vi "Send Control Drag Ended.vi"(0 "Message Enqueuer in":refnum<class "Message Enqueuer.lvclass">, 5 "CtlRef":refnum<vi>, 7 "Time":u32, 9 "Result":enum16{"Drop Cancel", "Drop Move", "Drop Copy"}(ring)) -> (4 "Filtered EventDataMessage":refnum<class "ControlDragEndedMsg.lvclass">, 15 "error out":errorcluster)   [LabVIEW 2020, in "MVA Framework.lvlib" / "ActorEvents.lvlib" / "ControlDragEndedMsg.lvclass"]
doc: "<License>\nCopyright © 2017 Composed Systems, LLC | All rights reserved\nwww.composed.io\n\nAuthor: Ethan Stern <ethan.stern@composed.io>\n\nThis software is provided \"AS IS\" WITHOUT WARRANTIES, either express or implied, AND IS FOR EDUCATIONAL PURPOSES ONLY.\n</License>"
uses:
  ControlDragEndedMsg.lvclass
  <vilib>/ActorFramework/Message Enqueuer/Message Enqueuer.lvclass
  ControlDragEndedMsg.lvclass/ControlDragEndedMsg.ctl
  EventDataMessage/EventDataMessage.lvclass/EventDataMessage.ctl
  <vilib>/ActorFramework/Message Enqueuer/Message Enqueuer.lvclass/Message Enqueuer.ctl
  <vilib>/ActorFramework/Message Enqueuer/Enqueue.vi
  <vilib>/Utility/error.llb/Clear Errors.vi
  EventDataMessage/EventDataMessage.lvclass
  C:/Program Files/National Instruments/LabVIEW 2020/vi.lib/ActorFramework/Message/Message.lvclass
  <vilib>/ActorFramework/Message Priority Queue/Priority Enqueue.vi
  IEventFilter/IEventFilter.lvclass
panel:
  in  "error in (no error)":errorcluster
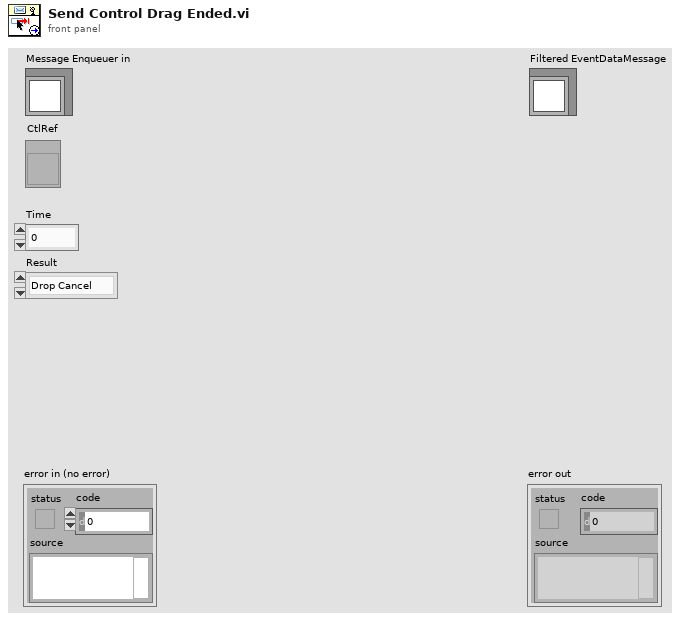
[diagram p1: front panel]
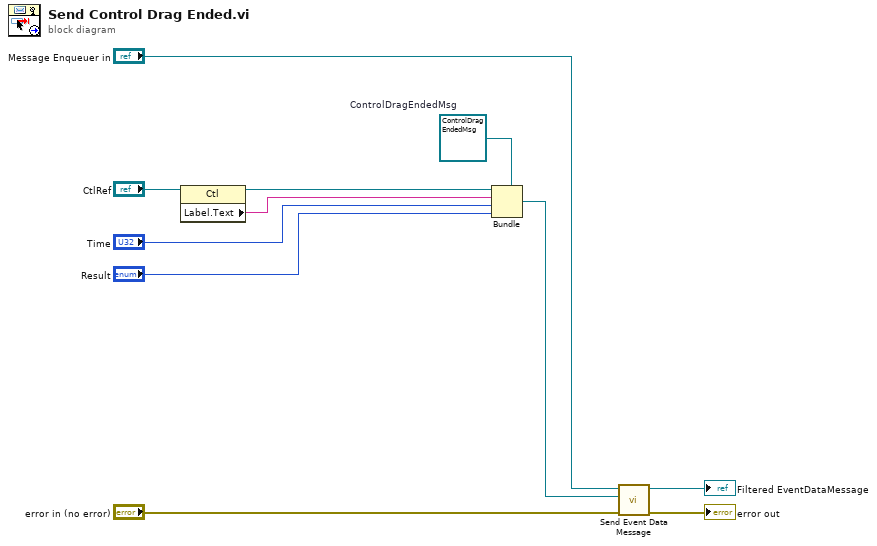
[diagram p0: block diagram]
diagram:
  w11 = refnum<class "ControlDragEndedMsg.lvclass"> refnum  # ControlDragEndedMsg
  n1 = property class="Ctl"(reference="CtlRef") -> (reference out=w5:refnum<vi>, "Label.Text"=w4:string)  [unwired: 1 in, 1 out]
  n2 = Bundle(cluster=w11, w5, w4, "Time", "Result") -> (w8:refnum<class "ControlDragEndedMsg.lvclass">)
  n3 = call "Send Event Data Message.vi"("error in (no error)"="error in (no error)", "EventDataMessage"=w8, "Message Enqueuer in"="Message Enqueuer in") -> ("error out"=→"error out":errorcluster, "Filtered EventDataMessage"=→"Filtered EventDataMessage":refnum<class "ControlDragEndedMsg.lvclass">)  [unwired: 7 in]
